vi "dfd_NPR Cosine-Modulated Prototype Filter Design.vi"(6 "weight":dbl=0.5, 7 "band counts":i32=4, 8 "error in (no error)":errorcluster, 10 "roll off":dbl=0.2, 11 "order":i32=38) -> (0 "error out":errorcluster, 3 "h":dbl[](array[numeric]))   [LabVIEW 2017, in "NI_DigFilter_FilterBank.lvlib"]
doc: "Designs the prototype filter of the Near-PR cosine modulated filter bank by optimizing the filter's coefficients to minimize the composite objective funtion of the stopband attenuation and the amplitude distortion."
uses:
  <vilib>/addons/Digital Filter Design/NI_DigFilter_FilterBank.lvlib
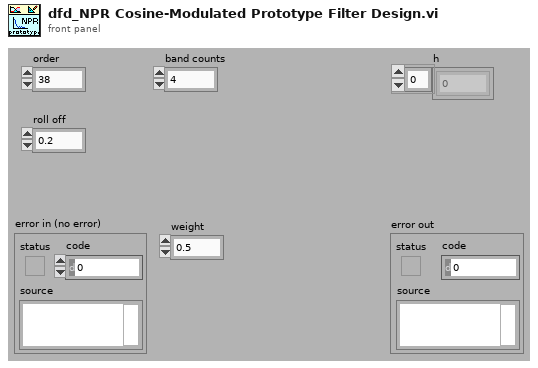
[diagram p1: front panel]
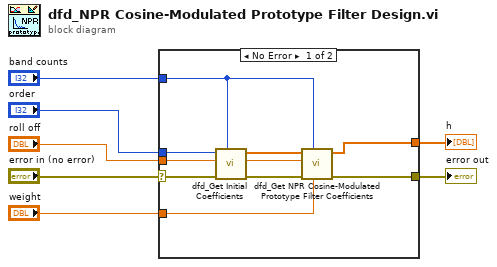
[diagram p0: block diagram]
diagram:
  n1 = case shown="No Error" "error in (no error)" {
    selector: "error in (no error)" -> [w17 w18]
    tunnel: [w15 _] -> w2
    tunnel: "weight" -> [w11 _]
    tunnel: "band counts" -> [w12 _]
    tunnel: [w16 w18] -> w7
    tunnel: "order" -> [w14 _]
    tunnel: "roll off" -> [w13 _]
    frame No Error {
      n2 = call <vilib>:"dfd_Get Initial Coefficients.vi"("M"=w12, "error in (no error)"=w17, "roll off"=w13, "order"=w14) -> ("error out"=w10:errorcluster, "dup roll off"=w9:dbl, "initial h"=w8:dbl[])  [unwired: 5 in]
      n3 = call <vilib>:"dfd_Get NPR Cosine-Modulated Prototype Filter Coefficients.vi"("gama"=w11, "number of bands"=w12, "error in (no error)"=w10, "roll off"=w9, "initial h"=w8) -> ("error out"=w16:errorcluster, "h"=w15:dbl[])  [unwired: 5 in]
    }
    frame Error {
    }
  }
  "h" <- w2
  "error out" <- w7
